vi "string array to csv.vi"(3 "String array":string[](array[string])) -> (1 "CSV":string)   [LabVIEW 2021, in "RocketPlot.lvlib"]
uses:
  RocketPlot.lvlib
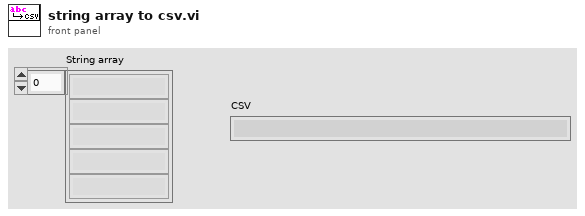
[diagram p1: front panel]
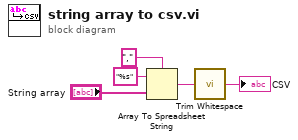
[diagram p0: block diagram]
diagram:
  n1 = Array To Spreadsheet String(delimiter (Tab)=",", array="String array", 3:"%s" ("format string")) -> (spreadsheet string=w2:string)
  n2 = call <vilib>:"Trim Whitespace.vi"("string"=w2) -> ("trimmed string"=→"CSV":string)  [unwired: 1 in]
